vi "Button Switch.vi"(8 "Right?":bool, 9 "Left?":bool, 10 "Bump Amount":dbl=1.0, 11 "Button in":bool) -> (0 "Right":bool, 1 "Left":bool, 3 "Bump":dbl)   [LabVIEW 2012]
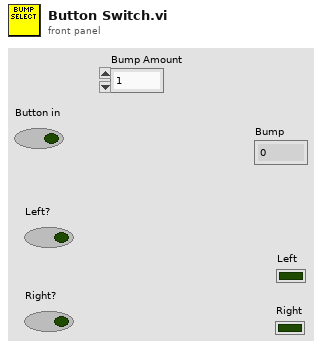
[diagram p1: front panel]
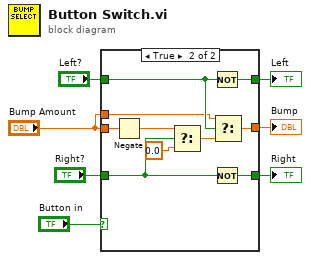
[diagram p0: block diagram]
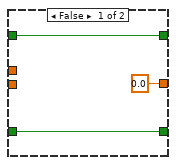
[diagram p2: hidden frame]
diagram:
  n1 = case shown="True" "Button in" {
    tunnel: "Left?" -> [w9 w15]
    tunnel: "Right?" -> [w10 w17]
    tunnel: [0.0 ("f") w18] -> w6
    tunnel: [w10 w16] -> w3
    tunnel: [w9 w14] -> w2
    tunnel: "Bump Amount" -> [_ w12]
    tunnel: "Bump Amount" -> [_ w11]
    frame False {
    }
    frame True {
      n2 = Negate(x=w12) -> (-x=w13:dbl)
      n3 = Select(t=w13, s=w17, f=0.0) -> (s? t:f=w20:dbl)
      n4 = Not(x=w15) -> (.not. x?=w14:bool)
      n5 = Not(x=w17) -> (.not. x?=w16:bool)
      n6 = Select(t=w11, s=w15, f=w20) -> (s? t:f=w18:dbl)
    }
  }
  "Left" <- w2
  "Bump" <- w6
  "Right" <- w3
